vi "Lifter SSS Tester.vi"() -> ()   [LabVIEW 2014]
uses:
  Subsystems VIs/Stacking SS/Stacking SS Actuators.ctl
  <vilib>/Rock Robotics/WPI/Solenoid/WPI_SolenoidValue.ctl
panel:
  in  "Bot":bool
  in  "TOp":bool
  in  "Lift Encoder":dbl(slide) scale=0.0..10.0
  in  "Time when Arm Last Moved":dbl format="%#_13g"
  out "Actuator Values Out":T1
  in  "Actuator Values in":T1
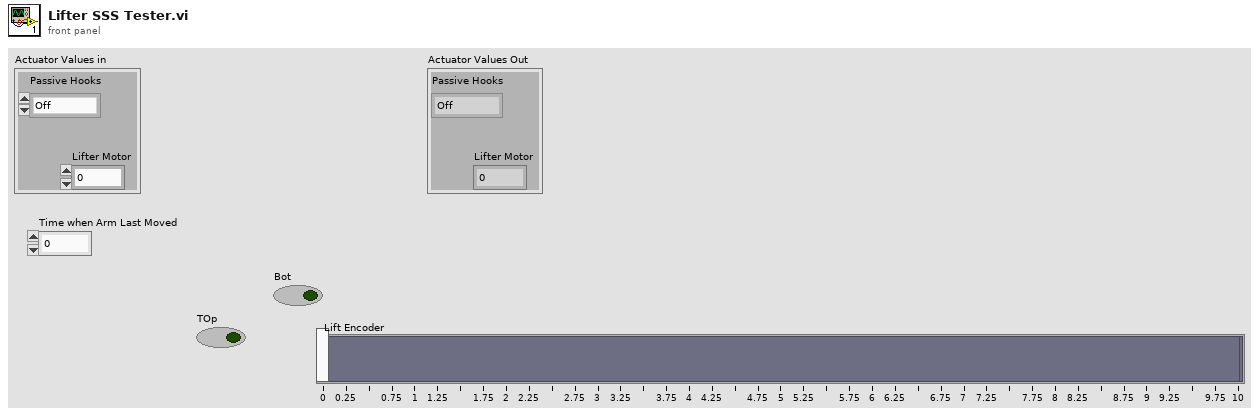
[diagram p1: front panel]
types:
  T1 = typedef "Stacking SS Actuators.ctl" = cluster{"Passive Hooks":T2, "Lifter Motor":dbl}
  T2 = typedef "WPI_SolenoidValue.ctl" = enum16{"Off", "On", "Forward", "Reverse"}
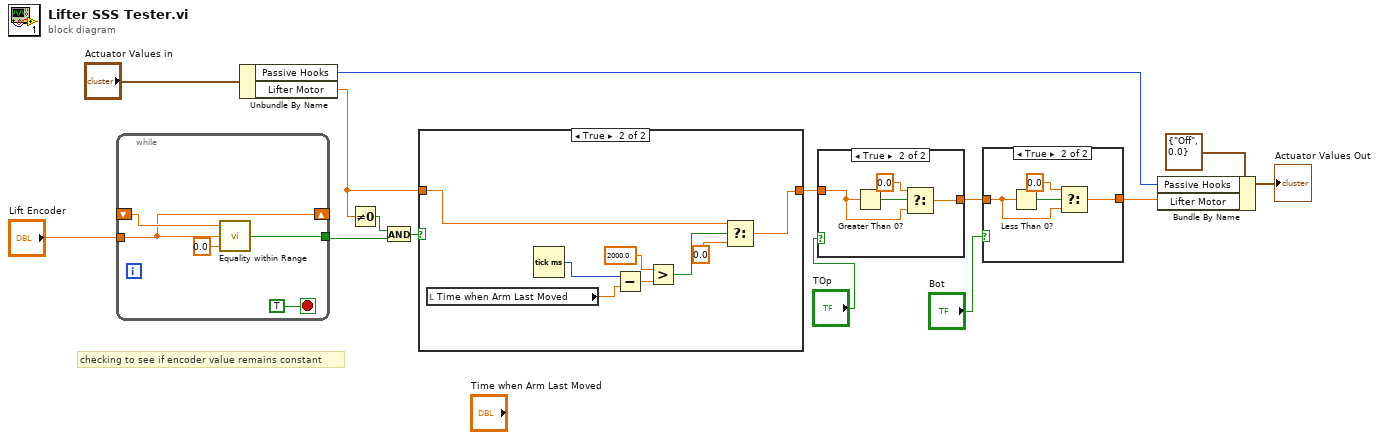
[diagram p0: block diagram]
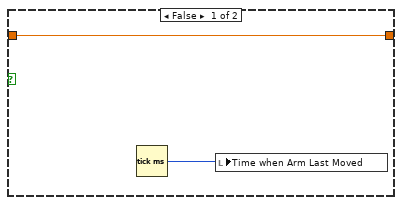
[diagram p2: hidden frame]
diagram:
  # "checking to see if encoder value remains constant"
  n1 = while {
    tunnel: [w15] -> w6
    shift-right: [w17] -> _
    shift-left: _ -> [w18]
    tunnel: "Lift Encoder" -> [w17]
    stop <- TRUE stop-if-true
    n2 = call "Equality within Range.vi"("Range"=0.0, "Y"=w17, "X"=w18) -> ("X = Y within Range?"=w15:bool)
  }
  n3 = Unbundle By Name("Actuator Values in") -> ("Passive Hooks"=w4:T2, "Lifter Motor"=w9:dbl)
  n4 = Not Equal To 0?(x=w9) -> (x != 0?=w7:bool)
  n5 = And(x=w7, y=w6) -> (x .and. y?=w8:bool)
  n6 = case shown="True" w8 {
    tunnel: w9 -> [w21 w25]
    tunnel: [w21 w24] -> w12
    frame False {
      n7 = Tick Count (ms)() -> (millisecond timer value=w20:u32)
      n8 = local write "Time when Arm Last Moved"(w20) -> ()
    }
    frame True {
      n9 = local read "Time when Arm Last Moved"() -> (w23:dbl)
      n10 = Tick Count (ms)() -> (millisecond timer value=w22:u32)
      n11 = Subtract(x=w22, y=w23) -> (x-y=w29:dbl)
      n12 = Greater?(x=2000.0, y=w29) -> (0:w26:bool)
      n13 = Select(t=w25, s=w26, f=0.0) -> (s? t:f=w24:dbl)
    }
  }
  n14 = case shown="True" "TOp" {
    tunnel: [w30 w33] -> w14
    tunnel: w12 -> [w30 w31]
    frame False {
    }
    frame True {
      n15 = Greater Than 0?(x=w31) -> (x > 0?=w34:bool)
      n16 = Select(t=0.0 ("f"), s=w34, f=w31) -> (s? t:f=w33:dbl)
    }
  }
  n17 = case shown="True" "Bot" {
    tunnel: w14 -> [w35 w36]
    tunnel: [w35 w38] -> w5
    frame False {
    }
    frame True {
      n18 = Less Than 0?(x=w36) -> (x < 0?=w39:bool)
      n19 = Select(t=0.0 ("f"), s=w39, f=w36) -> (s? t:f=w38:dbl)
    }
  }
  n20 = Bundle By Name(cluster=T1 {"Passive Hooks"=enum."Off", "Lifter Motor"=0.0} ("Actuator Values Out"), "Passive Hooks"=w4, "Lifter Motor"=w5) -> (→"Actuator Values Out":T1)
